vi "Digital Read.vi"   [LabVIEW 2013, in "LVH-LINX.lvlib"]
doc: "Read the value of the specified digital input channel(s)."
uses:
  <vilib>/LabVIEW Hacker/LINX/LVH-LINX.lvlib
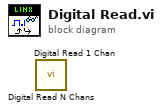
[diagram p0: block diagram]
diagram:
  n1 = call <vilib>:"Digital Read N Chans.vi"() -> ()  [unwired: 9 in, 3 out]
  n2 = call <vilib>:"Digital Read 1 Chan.vi"() -> ()  [unwired: 9 in, 3 out]
